vi "DriveBegin.vi"(8 "error in (no error)":errorcluster) -> (0 "error out":errorcluster)   [LabVIEW 2020]
doc: "Begin for Drive\n\nInputs:\n -- Error in -- Error cluster -- propagated error input\n\nOutputs:\n -- Error out -- Error cluster -- progated error output"
uses:
  <vilib>/Rock Robotics/WPI/ThirdParty/Phoenix-LabVIEW/Motor Controller/Controls/CTRE_Phoenix_MotorControl_NeutralMode.ctl
  <vilib>/Rock Robotics/WPI/Encoder/WPI_EncoderType.ctl
  <vilib>/Rock Robotics/SystemInterfaces/DIO/FPGA_DIOChannel.ctl
  <vilib>/Rock Robotics/WPI/Counter/WPI_CounterDigitalInputToDigitalSource.vi
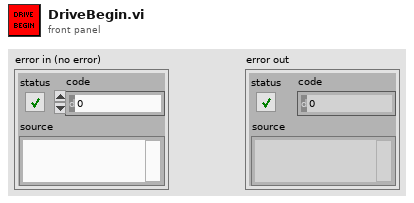
[diagram p1: front panel]
types:
  T1 = typedef "CTRE_Phoenix_MotorControl_NeutralMode.ctl" = enum8{"EEPROMSetting", "Override to Coast", "Override to Brake"}
  T2 = typedef "WPI_EncoderType.ctl" = enum16{"1x", "2x", "4x"}
  T3 = typedef "FPGA_DIOChannel.ctl" = enum8{"DIO 0", "DIO 1", "DIO 2", "DIO 3", "DIO 4", "DIO 5", "DIO 6", "DIO 7", "DIO 8", "DIO 9", "DIO MXP 0", "DIO MXP 1", "DIO MXP 2", "DIO MXP 3", "DIO MXP 4", "DIO MXP 5", "DIO MXP 6", "DIO MXP 7", "DIO MXP 8", "DIO MXP 9", "DIO MXP 10", "DIO MXP 11", "DIO MXP 12", "DIO MXP 13", "DIO MXP 14", "DIO MXP 15", "SPI Port CS1", "SPI Port CS2", "SPI Port CS3", "SPI Port MISO", "SPI Port MOSI", "Invalid"}
  T4 = typedef "WPI_MotorControlDeviceRef.ctl" = cluster{"DeviceStatus":errorcluster, "Type":T5, "PWM":cluster{"PWM Channel":T6, "DeadBand":T7}, "CAN":cluster{"Device Number":u8, "SetOutput VI Ref":variant, "GetOutput VI Ref":variant, "Enable VI Ref":variant, "Disable VI Ref":variant, "Data":variant}, "Invert":bool, "DIO PWM":cluster{"PWM \"Enable\" Channel":T6, "DIOChannel":T3, "PWM Rate":dbl}}
  T5 = typedef "WPI_MotorControlType.ctl" = enum16{"PWM", "CAN", "DIO PWM"}
  T6 = typedef "FPGA_DIOPWMChannel.ctl" = enum8{"PWM 0", "PWM 1", "PWM 2", "PWM 3", "PWM 4", "PWM 5", "PWM 6", "PWM 7", "PWM 8", "PWM 9", "PWM MXP 0", "PWM MXP 1", "PWM MXP 2", "PWM MXP 3", "PWM MXP 4", "PWM MXP 5", "PWM MXP 6", "PWM MXP 7", "PWM MXP 8", "PWM MXP 9", "Invalid"}
  T7 = typedef "WPI_PWMDeadband.ctl" = cluster{"Name":string, "maxPositivePwm":i32, "minPositivePwm":i32, "centerPwm":i32, "maxNegativePwm":i32, "minNegativePwm":i32, "angularRange":u16}
  T8 = typedef "WPI_DigitalInputDevRef.ctl" = cluster{"DevStatus":errorcluster, "DIO Channel":T3}
  T9 = typedef "ADIS16470 Device Reference.ctl" = cluster{"DevStatus":errorcluster, "Hardware Config":T10, "Calibration Complete":refnum<notifier>, "Status Reference":refnum<data-value>, "Data Reference":refnum<data-value>, "Sychronous Process VI":T13, "Cmd FIFO":refnum<k33>, "Source":T14, "Data FIFO":refnum<k33>, "Calibration Time (ms)":u32, "Data Reference":refnum<data-value>}
  T10 = typedef "ADIS16470 Hardware Configuration.ctl" = cluster{"SPI Clock Rate (Hz)":dbl, "IMU SPI Mode (3)":T11, "IMU Reset Pin":T3, "IMU SPI Bus":T12, "IMU Data Ready Pin":T3, "Stall Config":cluster{"Pow2BytesPerRead":u8, "StallTicks":u16, "CsToSclkTicks":u8}}
  T11 = typedef "WPI_SPIMode.ctl" = enum16{"Mode 0 (Clk Idle Low,Sample on Leading)", "Mode 1 (Clk Idle Low,Sample on Trailing)", "Mode 2 (Clk Idle High,Sample on Leading)", "Mode 3 (Clk Idle High,Sample on Trailing)"}
  T12 = typedef "spi_bus.ctl" = enum16{"SPI On-Board, CS0", "SPI On-Board, CS1", "SPI On-Board, CS2", "SPI On-Board, CS3", "SPI MXP", "Invalid"}
  T13 = typedef "ADIS16470 Process.ctl" = refnum<vi>
  T14 = typedef "FPGA_CounterEncoderSourceConvertionLVSourceType.ctl" = cluster{"DevStatus":errorcluster, "AnalogTriggerMode?":bool, "DigitalMode":cluster{"DIO Channel":T15}, "AnalogTriggerMode":cluster{"AnalogTriggerIndex":T16, "OutputType":T17}}
  T15 = typedef "FPGA_DIODigitalSourceChannel.ctl" = enum8{"DIO 0", "DIO 1", "DIO 2", "DIO 3", "DIO 4", "DIO 5", "DIO 6", "DIO 7", "DIO 8", "DIO 9", "DIO MXP 0", "DIO MXP 1", "DIO MXP 2", "DIO MXP 3", "DIO MXP 4", "DIO MXP 5", "DIO MXP 6", "DIO MXP 7", "DIO MXP 8", "DIO MXP 9", "DIO MXP 10", "DIO MXP 11", "DIO MXP 12", "DIO MXP 13", "DIO MXP 14", "DIO MXP 15", "SPI Port CS1", "SPI Port CS2", "SPI Port CS3", "SPI Port MISO", "SPI Port MOSI", "Disabled"}
  T16 = typedef "FPGA_AnalogTriggerIndex.ctl" = enum8{"Trig 0", "Trig 1", "Trig 2", "Trig 3", "Trig 4", "Trig 5", "Trig 6", "Trig 7", "Invalid"}
  T17 = typedef "FPGA_AnalogTriggerOutType.ctl" = enum16{"InWindow", "TriggerState", "Rising", "Falling"}
  T18 = typedef "WPI_EncoderDevRef.ctl" = cluster{"DevStatus":errorcluster, "EncoderIndex":T19, "CounterIndex":T20, "DistancePerCount":dbl, "Decoding Type":T2}
  T19 = typedef "FPGA_EncoderIdx.ctl" = enum8{"Enc 0", "Enc 1", "Enc 2", "Enc 3", "Enc 4", "Enc 5", "Enc 6", "Enc 7", "Invalid"}
  T20 = typedef "FPGA_CounterCtrSystemIndex.ctl" = enum8{"Ctr 0", "Ctr 1", "Ctr 2", "Ctr 3", "Ctr 4", "Ctr 5", "Ctr 6", "Ctr 7", "Invalid"}
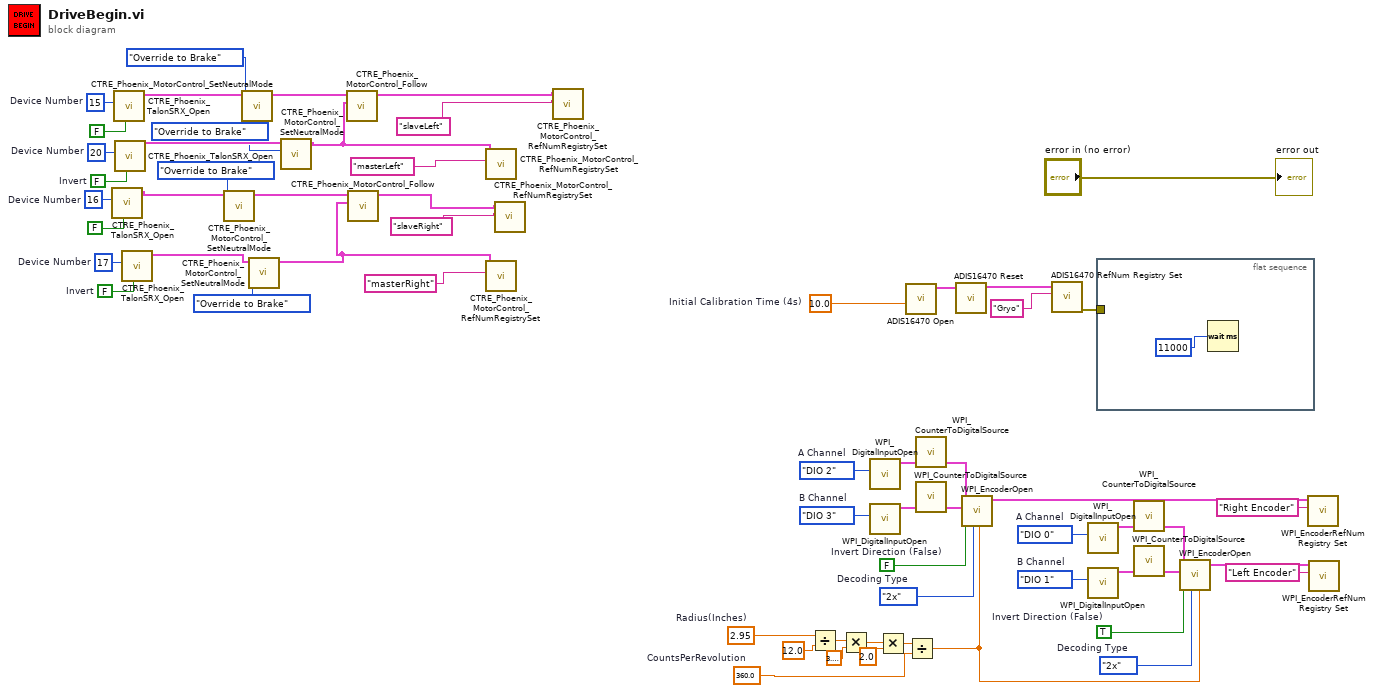
[diagram p0: block diagram]
diagram:
  w3 = u8 16  # Device Number
  w4 = u8 15  # Device Number
  w24 = 10.0  # Initial Calibration Time (4s)
  w30 = TRUE  # Invert Direction (False)
  w31 = WPI_EncoderType."2x"  # Decoding Type
  w33 = FALSE  # Invert Direction (False)
  w34 = WPI_EncoderType."2x"  # Decoding Type
  w35 = 360.0  # CountsPerRevolution
  w39 = 2.95  # Radius(Inches)
  w46 = FPGA_DIOChannel."DIO 1"  # B Channel
  w45 = FPGA_DIOChannel."DIO 0"  # A Channel
  w52 = FPGA_DIOChannel."DIO 3"  # B Channel
  w51 = FPGA_DIOChannel."DIO 2"  # A Channel
  w55 = FALSE  # Invert
  w56 = FALSE  # Invert
  w58 = u8 17  # Device Number
  w57 = u8 20  # Device Number
  n1 = call <vilib>:"CTRE_Phoenix_TalonSRX_Open.vi"("Invert"=FALSE, "Device Number"=w3) -> ("PhoenixMotorControlDevRef"=w10:T4)  [unwired: 8 in, 1 out]
  n2 = call <vilib>:"CTRE_Phoenix_TalonSRX_Open.vi"("Invert"=FALSE, "Device Number"=w4) -> ("PhoenixMotorControlDevRef"=w16:T4)  [unwired: 8 in, 1 out]
  n3 = call <vilib>:"CTRE_Phoenix_TalonSRX_Open.vi"("Invert"=w55, "Device Number"=w57) -> ("PhoenixMotorControlDevRef"=w19:T4)  [unwired: 8 in, 1 out]
  n4 = call <vilib>:"CTRE_Phoenix_TalonSRX_Open.vi"("Invert"=w56, "Device Number"=w58) -> ("PhoenixMotorControlDevRef"=w21:T4)  [unwired: 8 in, 1 out]
  n5 = call <vilib>:"CTRE_Phoenix_MotorControl_SetNeutralMode.vi"("Motor Control Neutral Mode"=CTRE_Phoenix_MotorControl_NeutralMode."Override to Brake", "PhoenixMotorControlDevRef"=w10) -> ("PhoenixMotorControlDevRef"=w9:T4)  [unwired: 8 in, 1 out]
  n6 = call <vilib>:"CTRE_Phoenix_MotorControl_SetNeutralMode.vi"("Motor Control Neutral Mode"=CTRE_Phoenix_MotorControl_NeutralMode."Override to Brake", "PhoenixMotorControlDevRef"=w16) -> ("PhoenixMotorControlDevRef"=w14:T4)  [unwired: 8 in, 1 out]
  n7 = call <vilib>:"CTRE_Phoenix_MotorControl_SetNeutralMode.vi"("Motor Control Neutral Mode"=CTRE_Phoenix_MotorControl_NeutralMode."Override to Brake", "PhoenixMotorControlDevRef"=w21) -> ("PhoenixMotorControlDevRef"=w8:T4)  [unwired: 8 in, 1 out]
  n8 = call <vilib>:"CTRE_Phoenix_MotorControl_SetNeutralMode.vi"("Motor Control Neutral Mode"=CTRE_Phoenix_MotorControl_NeutralMode."Override to Brake", "PhoenixMotorControlDevRef"=w19) -> ("PhoenixMotorControlDevRef"=w13:T4)  [unwired: 8 in, 1 out]
  n9 = call <vilib>:"CTRE_Phoenix_MotorControl_Follow.vi"("Master Controller to Follow"=w13, "PhoenixMotorControlDevRef"=w14) -> ("PhoenixMotorControlDevRef"=w12:T4)  [unwired: 8 in, 1 out]
  n10 = call <vilib>:"CTRE_Phoenix_MotorControl_Follow.vi"("Master Controller to Follow"=w8, "PhoenixMotorControlDevRef"=w9) -> ("PhoenixMotorControlDevRef"=w7:T4)  [unwired: 8 in, 1 out]
  n11 = call <vilib>:"CTRE_Phoenix_MotorControl_RefNumRegistrySet.vi"("refnum name"="masterLeft", "PhoenixMotorControlDevRef"=w13) -> ()  [unwired: 8 in, 2 out]
  n12 = call <vilib>:"CTRE_Phoenix_MotorControl_RefNumRegistrySet.vi"("refnum name"="masterRight", "PhoenixMotorControlDevRef"=w8) -> ()  [unwired: 8 in, 2 out]
  n13 = call <vilib>:"CTRE_Phoenix_MotorControl_RefNumRegistrySet.vi"("refnum name"="slaveRight", "PhoenixMotorControlDevRef"=w7) -> ()  [unwired: 8 in, 2 out]
  n14 = call <vilib>:"CTRE_Phoenix_MotorControl_RefNumRegistrySet.vi"("refnum name"="slaveLeft", "PhoenixMotorControlDevRef"=w12) -> ()  [unwired: 8 in, 2 out]
  n15 = Divide(x=w39, y=12.0) -> (x/y=w38:dbl)
  n16 = Multiply(x=w38, y=3.141592653589793) -> (x*y=w41:dbl)
  n17 = call <vilib>:"WPI_DigitalInputOpen.vi"("DIO Channel"=w51) -> ("DigitalInputDevRef"=w49:T8)  [unwired: 1 in, 9 out]
  n18 = call <vilib>:"WPI_DigitalInputOpen.vi"("DIO Channel"=w52) -> ("DigitalInputDevRef"=w50:T8)  [unwired: 1 in, 9 out]
  n19 = Multiply(x=w41, y=2.0) -> (x*y=w42:dbl)
  n20 = call <vilib>:"ADIS16470 Open.vi"("Initial Calibration Time (4s)"=w24) -> ("ADIS16470DevRef"=w23:T9)  [unwired: 9 in, 1 out]
  n21 = Divide(x=w42, y=w35) -> (x/y=w32:dbl)
  n22 = call-poly <vilib>:"WPI_CounterToDigitalSource.vi"("DigitalInputDevRef"=w49) -> ("Digital Source"=w53:T14)  [unwired: 6 out]
  n23 = call-poly <vilib>:"WPI_CounterToDigitalSource.vi"("DigitalInputDevRef"=w50) -> ("Digital Source"=w54:T14)  [unwired: 6 out]
  n24 = call <vilib>:"ADIS16470 Reset.vi"("ADIS16470DevRef"=w23) -> ("ADIS16470DevRef"=w22:T9)  [unwired: 9 in, 1 out]
  n25 = call <vilib>:"WPI_EncoderOpen.vi"("DistancePerCount"=w32, "Decoding Type"=w34, "Invert Direction (False)"=w33, "BSource"=w54, "ASource"=w53) -> ("EncoderDevRef"=w29:T18)  [unwired: 5 in, 1 out]
  n26 = call <vilib>:"ADIS16470 RefNum Registry Set.vi"("refnum name"="Gryo", "ADIS16470DevRef in"=w22) -> ("error out"=w17:errorcluster)  [unwired: 8 in, 1 out]
  n27 = call <vilib>:"WPI_DigitalInputOpen.vi"("DIO Channel"=w45) -> ("DigitalInputDevRef"=w43:T8)  [unwired: 1 in, 9 out]
  n28 = call <vilib>:"WPI_DigitalInputOpen.vi"("DIO Channel"=w46) -> ("DigitalInputDevRef"=w44:T8)  [unwired: 1 in, 9 out]
  n29 = flat-sequence {
    tunnel: w17 -> [_]
    frame #0 {
      n30 = Wait (ms)(milliseconds to wait=u32 11000) -> ()  [unwired: 1 out]
    }
  }
  n31 = call-poly <vilib>:"WPI_CounterToDigitalSource.vi"("DigitalInputDevRef"=w43) -> ("Digital Source"=w47:T14)  [unwired: 6 out]
  n32 = call-poly <vilib>:"WPI_CounterToDigitalSource.vi"("DigitalInputDevRef"=w44) -> ("Digital Source"=w48:T14)  [unwired: 6 out]
  n33 = call <vilib>:"WPI_EncoderOpen.vi"("DistancePerCount"=w32, "Decoding Type"=w31, "Invert Direction (False)"=w30, "BSource"=w48, "ASource"=w47) -> ("EncoderDevRef"=w26:T18)  [unwired: 5 in, 1 out]
  n34 = call <vilib>:"WPI_EncoderRefNum Registry Set.vi"("refnum name"="Right Encoder", "EncoderDevRef"=w29) -> ()  [unwired: 8 in, 2 out]
  n35 = call <vilib>:"WPI_EncoderRefNum Registry Set.vi"("refnum name"="Left Encoder", "EncoderDevRef"=w26) -> ()  [unwired: 8 in, 2 out]
  "error out" <- "error in (no error)"
